vi "Ping.vi"(8 "error in":errorcluster, 10 "timeout":i32=1000, 11 "hostNameOrAddress":string="127.0.0.1") -> (0 "error out":errorcluster, 3 "Ping Status":bool)   [LabVIEW 2021]
panel:
  out "Ping Error":errorcluster
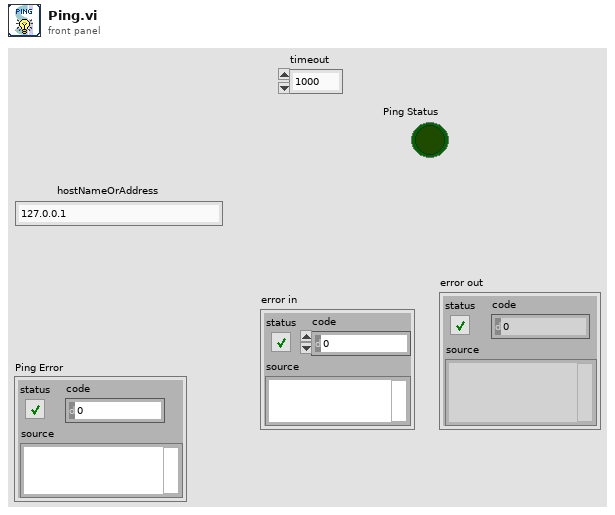
[diagram p1: front panel]
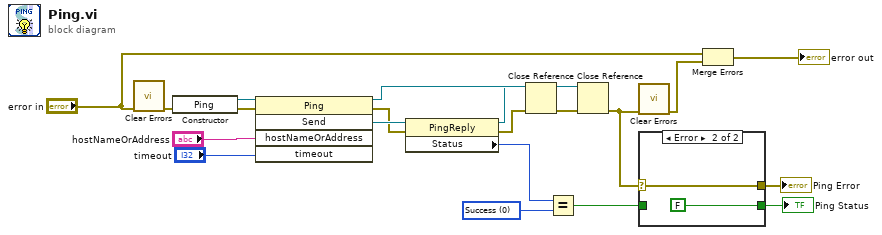
[diagram p0: block diagram]
diagram:
  w14 = 0 items=["Success"=0, "DestinationNetworkUnreachable"=11002, "DestinationHostUnreachable"=11003, "DestinationProhibited, DestinationProtocolUnreachable"=11004, "DestinationPortUnreachable"=11005, "NoResources"=11006, "BadOption"=11007, "HardwareError"=11008, "PacketTooBig"=11009, "TimedOut"=11010, "BadRoute"=11012, "TtlExpired"=11013, "TtlReassemblyTimeExceeded"=11014, "ParameterProblem"=11015, "SourceQuench"=11016, "BadDestination"=11018, "DestinationUnreachable"=11040, "TimeExceeded"=11041, "BadHeader"=11042, "UnrecognizedNextHeader"=11043, "IcmpError"=11044, "DestinationScopeMismatch"=11045, "Unknown"=-1] ("Status")
  n1 = call <vilib>:"Clear Errors.vi"("error in (no error)"="error in") -> ("error out"=w4:errorcluster)  [unwired: 5 in, 1 out]
  n2 = constructor class="Ping"(error in=w4) -> (reference out=w20:refnum<k24>, error out=w19:errorcluster)  [unwired: 2 in, 1 out]
  n3 = invoke class="Ping" method="Send"(reference=w20, error in=w19, "hostNameOrAddress"="hostNameOrAddress", "timeout"="timeout") -> (reference out=w17:refnum<k24>, error out=w16:errorcluster, "Send"=w18:refnum<k24>)  [unwired: 1 in, 2 out]
  n4 = property class="PingReply"(reference=w18, error in=w16) -> (reference out=w15:refnum<k24>, error out=w12:errorcluster, "Status"=w13:i32)
  n5 = Close Reference(reference=w17, error in (no error)=w12) -> (error out=w11:errorcluster)
  n6 = Equal?(x=w13, y=w14) -> (x = y?=w9:bool)
  n7 = Close Reference(reference=w15, error in (no error)=w11) -> (error out=w10:errorcluster)
  n8 = call <vilib>:"Clear Errors.vi"("error in (no error)"=w10) -> ("error out"=w7:errorcluster)  [unwired: 5 in, 1 out]
  n9 = case shown="Error" w10 {
    selector: w10 -> [w21 w23]
    tunnel: w9 -> [w22 _]
    tunnel: [w22 FALSE] -> w8
    tunnel: [w21 w23] -> w1
    frame No Error {
    }
    frame Error {
    }
  }
  "Ping Status" <- w8
  "Ping Error" <- w1
  n10 = Merge Errors("error in", w7) -> (→"error out":errorcluster)
